vi "Meas Result Readings Panel.vi"(8 "error in":errorcluster, 11 "meas in":variant) -> (0 "error out":errorcluster, 3 "meas out":variant)   [LabVIEW 2020]
doc: "Panel for manual removal of readings."
uses:
  meas session.ctl
  Meas Sweep Config.ctl
  Meas Freq Info.ctl
  meas_swp_mode.ctl
  meas_sweep_flist_mode.ctl
  bridge/Bridge Session.ctl
  bridge/Bridge Type.ctl
  drivers/TWM client/TWM Session.ctl
  drivers/TWM client/TWM parameters.ctl
  drivers/TWM client/Meas Proc QWTB Uncertainty Mode.ctl
  bridge/Bridge Bias Session.ctl
  bridge/Bridge Bias Type.ctl
  bridge/Bridge Sim Mode.ctl
  source/Source Session.ctl
  source/Source Type.ctl
  drivers/AFG3101C/AFG3101C Session.ctl
  drivers/cDAQ DDS/cDAQ DDS Session.ctl
  drivers/cDAQ DDS/cDAQ DDS Setup.ctl
  drivers/cDAQ DDS/cDAQ DDS Timebase Mode.ctl
  drivers/Fluke 5XXX/top_lev/F5xxx_session.ctl
  drivers/Fluke 5XXX/top_lev/F5xxx_output_mode.ctl
  Meas Results Ref.ctl
  Meas Results.ctl
  bridge/Bridge Frequency Readings Data.ctl
  drivers/TWM client/Meas Proc QWTB Spectrum Data.ctl
  drivers/TWM client/TWM Phase Info.ctl
  Meas Result Major Format.ctl
  varilib/SGUI Assign References Mode.ctl
  <vilib>/Utility/miscctls.llb/LVRowAndColumnTypeDef.ctl
  varilib/varilib.lvlib
panel:
  in  "table xls":string[][](table) caption="Readings"
  in  "mnr fmt":T1=enum."%_5p" caption="Minor format"
  in  "mjr fmt":T1=enum."%_5p" caption="Major format"
  out "sweep spot index":u16
  out "phase index":u16
  in  "meas in":T2={"swp cfg"={"N"=0, "R"=0, "f list"=[], "smpl delay"=0.0, "set delay"=0.0, "set delay np"=0.0, "meas root"=path "", "meas name"="", "meas a-index"=FALSE, "rnd sweep"=FALSE, "mode"=enum."Frequency", "swp mode"=enum."Linear", "avg"=0, "subrec"=0, "multi-freq"=FALSE, "selfcal"=FALSE, "selfcal period [h]"=0.0}, "bridge"={"type"=enum."TWM client", "TWM"={"pipe name"="", "parameters"=[], "handle"=0, "fixed aper [s]"=0.0, "f-list [Hz]"=[], "discrete f-list"=FALSE, "unc mode"=enum."None", "unc mcc"=0, "unc first"=FALSE}, "last f"=0.0, "bias comp"={"bias type"=enum."dummy", "VISA"="", "Enable"=FALSE, "channel qu"=[], "channel Uinit"=[]}, "sim mode"=enum."Generic RLC network", "channel idns"=[], "sim phases"=1}, "src"={"type"=enum."Tektronix AFG3101C", "afg"={"VISA"="", "const"=0.0, "gen DC"=FALSE, "ext ref"=FALSE}, "cDAQ dds"={"device"="", "channels"=[], "mclk source"="", "mclk [Hz]"=0.0, "fs [Hz]"=0.0, "block [s]"=0.0, "buf [s]"=0.0, "task"="", "cmd queue"=refnum, "proc ref"=refnum, "smpl clock out"="/cDAQ3/PFI0", "export smpl clock"=FALSE, "DC ofs [V]"=[], "timebase source"="", "timebase mode"=enum."Local"}, "gain [V/A]"=1.0, "F5xxx session"={"VISA"="", "mode"=enum."AC voltage", "Earth on"=FALSE, "Ext ref lock"=FALSE}}, "results"=refnum} {"src"."cDAQ dds"."channels" min=0 step=1; "bridge"."TWM"."f-list [Hz]" format="%#_6p"; "swp cfg"."f list"."bias" format="%#_3p"; "swp cfg"."f list"."level" format="%#_3p"; "swp cfg"."f list"."fs [Hz]" format="%#_5p"; "swp cfg"."f list"."time [s]" format="%#_3p"; "swp cfg"."f list"."f/fs" format="%#_3p"; "swp cfg"."f list"."periods" format="%#_3f"; "swp cfg"."f list"."f [Hz]" format="%#_5p"}
  in  "btn rem":bool
  in  "rdgs ring spot":u16(ring) caption="Sweep spot selection" items=["Last measured"]
  in  "rdgs ring phase":u16(ring) caption="Phase selection"
  in  "btn ok":bool
  in  "table":string[][](table) caption="Readings (right click to show actions)"
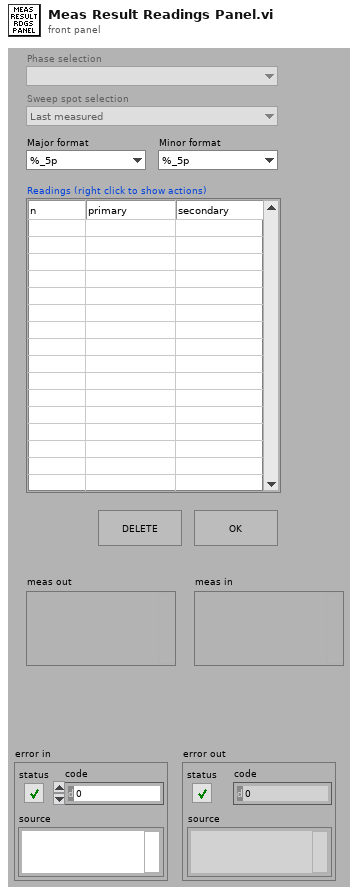
[diagram p1: front panel]
types:
  T1 = typedef "Meas Result Major Format.ctl" = enum16{"%_3p", "%_4p", "%_5p", "%_6p", "%_7p", "%_8p", "%_5f", "%_6f", "%_7f", "%_8f", "%_5e", "%_6e", "%_7e", "%_8e"}
  T2 = typedef "meas session.ctl" = cluster{"swp cfg":T3, "bridge":T7, "src":T15, "results":T22}
  T3 = typedef "Meas Sweep Config.ctl" = cluster{"N":i32, "R":i32, "f list":T4[], "smpl delay":dbl, "set delay":dbl, "set delay np":dbl, "meas root":path, "meas name":string, "meas a-index":bool, "rnd sweep":bool, "mode":T5, "swp mode":T6, "avg":i32, "subrec":i32, "multi-freq":bool, "selfcal":bool, "selfcal period [h]":dbl}
  T4 = typedef "Meas Freq Info.ctl" = cluster{"f [Hz]":dbl, "periods":dbl, "f/fs":dbl, "time [s]":dbl, "fs [Hz]":dbl, "N":i32, "level":dbl, "bias":dbl, "rdgs":i32, "f. id":i32}
  T5 = typedef "meas_swp_mode.ctl" = enum16{"Frequency", "Level", "Bias"}
  T6 = typedef "meas_sweep_flist_mode.ctl" = enum16{"Linear", "Log10"}
  T7 = typedef "Bridge Session.ctl" = cluster{"type":T8, "TWM":T9, "last f":dbl, "bias comp":T12, "sim mode":T14, "channel idns":string[], "sim phases":i32}
  T8 = typedef "Bridge Type.ctl" = enum16{"TWM client", "dummy"}
  T9 = typedef "TWM Session.ctl" = cluster{"pipe name":string, "parameters":T10[], "handle":i32, "fixed aper [s]":dbl, "f-list [Hz]":dbl[], "discrete f-list":bool, "unc mode":T11, "unc mcc":i32, "unc first":bool}
  T10 = typedef "TWM parameters.ctl" = cluster{"name":string, "value":string[]}
  T11 = typedef "Meas Proc QWTB Uncertainty Mode.ctl" = enum16{"None", "GUF", "Monte Carlo"}
  T12 = typedef "Bridge Bias Session.ctl" = cluster{"bias type":T13, "VISA":refnum<visa-resource-name>, "Enable":bool, "channel qu":string[], "channel Uinit":dbl[]}
  T13 = typedef "Bridge Bias Type.ctl" = enum16{"dummy", "CMI LiBbias V1.0"}
  T14 = typedef "Bridge Sim Mode.ctl" = enum16{"Generic RLC network", "Interchannel transfer"}
  T15 = typedef "Source Session.ctl" = cluster{"type":T16, "afg":T17, "cDAQ dds":T18, "gain [V/A]":dbl, "F5xxx session":T20}
  T16 = typedef "Source Type.ctl" = enum16{"Tektronix AFG3101C", "cDAQ DAC", "Fluke 5xxx", "Agilent 33120A", "dummy"}
  T17 = typedef "AFG3101C Session.ctl" = cluster{"VISA":refnum<visa-resource-name>, "const":dbl, "gen DC":bool, "ext ref":bool}
  T18 = typedef "cDAQ DDS Session.ctl" = cluster{"device":tag, "channels":i32[], "mclk source":tag, "mclk [Hz]":dbl, "fs [Hz]":dbl, "block [s]":dbl, "buf [s]":dbl, "task":refnum<k21>, "cmd queue":refnum<queue>, "proc ref":refnum<vi>, "smpl clock out":tag, "export smpl clock":bool, "DC ofs [V]":dbl[], "timebase source":tag, "timebase mode":T19}
  T19 = typedef "cDAQ DDS Timebase Mode.ctl" = enum16{"Local", "Take from ADC (e.g. NI 9238)", "Other source"}
  T20 = typedef "F5xxx_session.ctl" = cluster{"VISA":refnum<visa-resource-name>, "mode":T21, "Earth on":bool, "Ext ref lock":bool}
  T21 = typedef "F5xxx_output_mode.ctl" = enum16{"AC voltage", "AC current"}
  T22 = typedef "Meas Results Ref.ctl" = refnum<vi>
  T23 = typedef "varilib.lvlib/SGUI Assign References Mode.ctl" = enum16{"Add to stack", "Overwrite", "Release last", "Release ID"}
  T24 = typedef "LVRowAndColumnTypeDef.ctl" = cluster{"Row":i32, "Column":i32}
  T25 = typedef "Meas Results.ctl" = cluster{"freqs":T26[][], "locked":bool, "last fid":i32, "modified":bool, "mjr name":string, "mnr name":string, "last spectra":T27[][], "saved?":bool, "TWM phase":T28[], "time start":timestamp, "time stop":timestamp}
  T26 = typedef "Bridge Frequency Readings Data.ctl" = cluster{"Udut":dbl[], "Iref":dbl[], "Udc":dbl[], "Idc":dbl[], "mjr":dbl[], "mnr":dbl[], "mjr_sh":dbl[], "mnr_sh":dbl[], "u(mjr)":dbl[], "u(mnr)":dbl[], "ua2(mjr)":dbl[], "ua2(mnr)":dbl[], "n":i32, "f [Hz]":dbl, "fs [Hz]":dbl, "aperture [s]":dbl}
  T27 = typedef "Meas Proc QWTB Spectrum Data.ctl" = cluster{"x":sgl[], "y":sgl[], "label":string}
  T28 = typedef "TWM Phase Info.ctl" = cluster{"ref chn id (I)":string, "dut chn id (U)":string, "ref chn range [V]":dbl, "dut chn range [V]":dbl, "aperture [s]":dbl, "fs [Hz]":dbl, "ref chn transducer (I)":string, "dut chn transducer (U)":string}
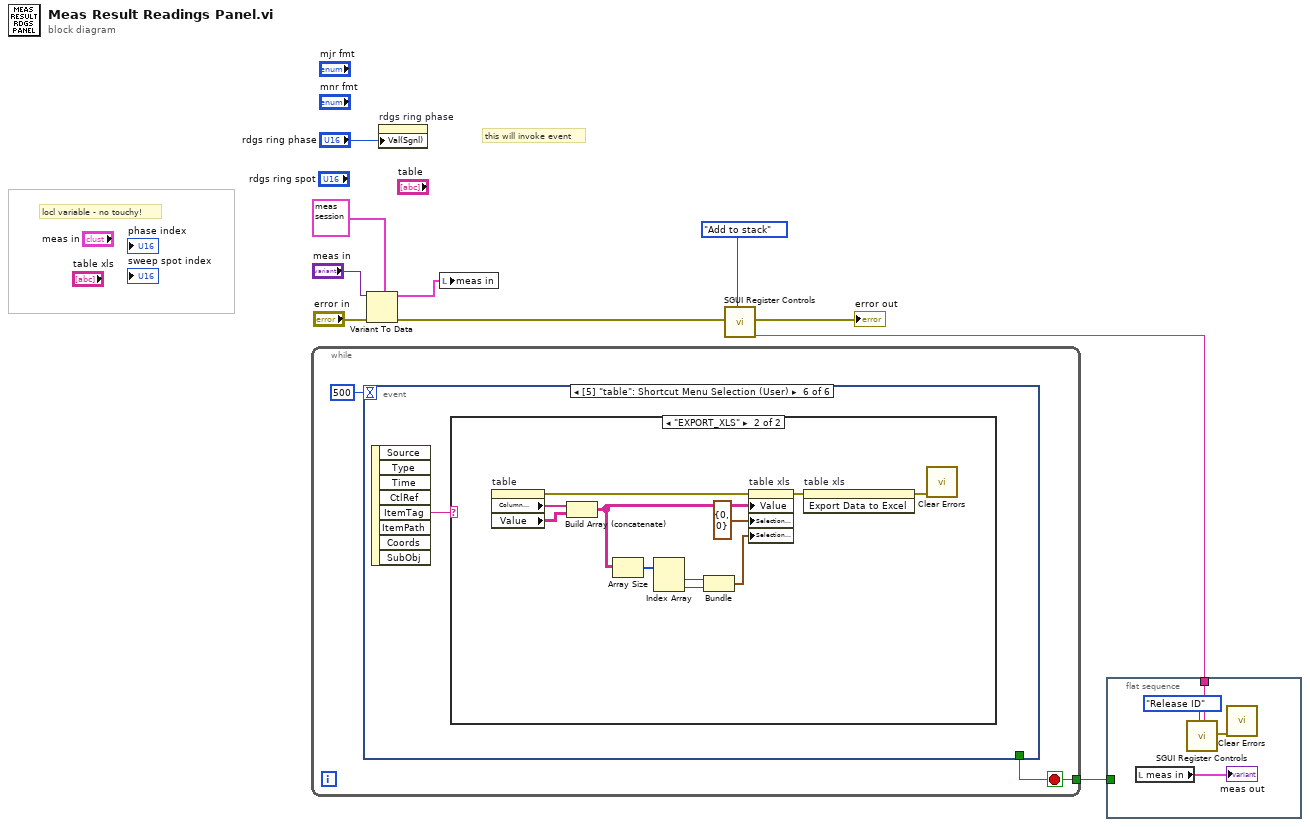
[diagram p0: block diagram]
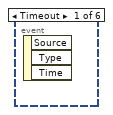
[diagram p2: hidden frame]
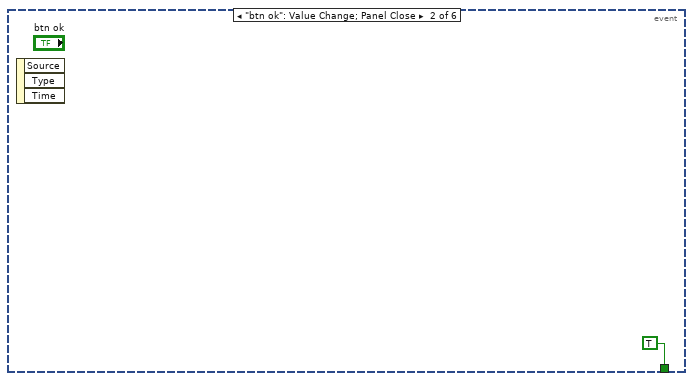
[diagram p3: hidden frame]
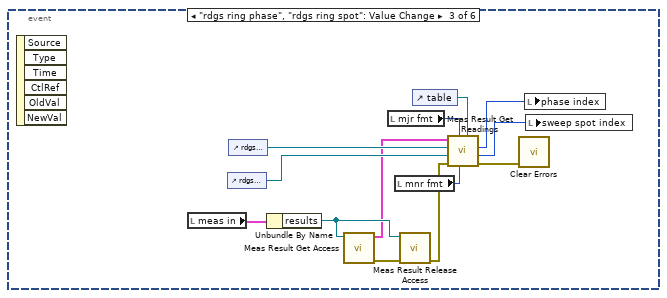
[diagram p4: hidden frame]
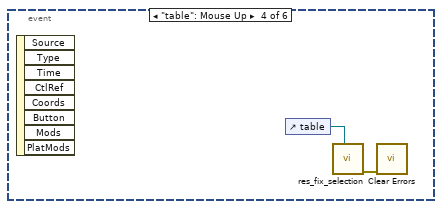
[diagram p5: hidden frame]
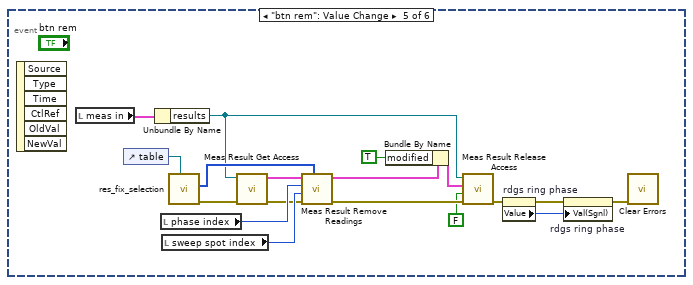
[diagram p6: hidden frame]
diagram:
  # "locl variable - no touchy!"
  # "this will invoke event"
  n1 = while {
    tunnel: [w12] -> w5
    stop <- w12 stop-if-true
    n2 = event shown="[5] \"table\": Shortcut Menu Selection (User)" {
      selector: _ -> [_ _ _ _ _ _]
      dyn-events: _ -> [_ _ _ _ _ _]
      timeout: 500 -> [_ _ _ _ _ _]
      tunnel: [_ TRUE _ _ _ _] -> w12
      event Timeout {
        n3 = event-data() -> ()  [unwired: 1 in, 3 out]
      }
      event "btn ok": Value Change; Panel Close {
        n4 = event-data() -> ()  [unwired: 1 in, 3 out]
      }
      event "rdgs ring phase", "rdgs ring spot": Value Change {
        n5 = event-data() -> ()  [unwired: 1 in, 6 out]
        n6 = local read "meas in"() -> (w22:T2)
        n7 = control-ref of="rdgs ring spot"() -> (w25:refnum<vi>)
        n8 = control-ref of="rdgs ring phase"() -> (w26:refnum<vi>)
        n9 = Unbundle By Name(w22) -> ("results"=w23:T22)
        n10 = call "Meas Result Get Access.vi"("results ref"=w23) -> ("error out"=w24:errorcluster, "results data"=w21:T25)  [unwired: 9 in]
        n11 = local read "mjr fmt"() -> (w15:T1)
        n12 = local read "mnr fmt"() -> (w14:T1)
        n13 = call "Meas Result Release Access.vi"("error in"=w24, "results ref"=w23) -> ("error out"=w19:errorcluster)  [unwired: 9 in]
        n14 = control-ref of="table"() -> (w20:refnum<vi>)
        n15 = call "Meas Result Get Readings.vi"("table ref"=w20, "mnr fmt"=w14, "mjr fmt"=w15, "error in (no error)"=w19, "ring spot"=w25, "ring phase"=w26, "result"=w21) -> ("error out"=w18:errorcluster, "sweep spot index"=w16:u16, "phase index"=w17:u16)  [unwired: 2 out]
        n16 = call <vilib>:"Clear Errors.vi"("error in (no error)"=w18) -> ()  [unwired: 5 in, 2 out]
        n17 = local write "phase index"(w17) -> ()
        n18 = local write "sweep spot index"(w16) -> ()
      }
      event "table": Mouse Up {
        n19 = event-data() -> ()  [unwired: 1 in, 8 out]
        n20 = control-ref of="table"() -> (w28:refnum<vi>)
        n21 = call "res_fix_selection.vi"("list"=w28) -> ("error out"=w27:errorcluster)  [unwired: 8 in, 2 out]
        n22 = call <vilib>:"Clear Errors.vi"("error in (no error)"=w27) -> ()  [unwired: 5 in, 2 out]
      }
      event "btn rem": Value Change {
        n23 = event-data() -> ()  [unwired: 1 in, 6 out]
        n24 = local read "meas in"() -> (w39:T2)
        n25 = control-ref of="table"() -> (w40:refnum<vi>)
        n26 = Unbundle By Name(w39) -> ("results"=w37:T22)
        n27 = local read "phase index"() -> (w46:u16)
        n28 = local read "sweep spot index"() -> (w45:u16)
        n29 = call "res_fix_selection.vi"("list"=w40) -> ("error out"=w44:errorcluster, "ids of selected"=w38:i32[])  [unwired: 8 in, 1 out]
        n30 = call "Meas Result Get Access.vi"("error in"=w44, "results ref"=w37) -> ("error out"=w43:errorcluster, "results data"=w42:T25)  [unwired: 8 in]
        n31 = call "Meas Result Remove Readings.vi"("ids of selected"=w38, "error in"=w43, "sweep spot index"=w45, "phase index"=w46, "result"=w42) -> ("error out"=w41:errorcluster, "result out"=w31:T25)  [unwired: 5 in]
        n32 = Bundle By Name(cluster=w31, "modified"=TRUE) -> (w30:T25)
        n33 = call "Meas Result Release Access.vi"("error in"=w41, "Release only (True)"=FALSE, "results data in"=w30, "results ref"=w37) -> ("error out"=w35:errorcluster)  [unwired: 7 in]
        n34 = property on="rdgs ring phase" class="Ring (strict)"(error in=w35) -> (error out=w33:errorcluster, "Value"=w34:u16)  [unwired: 1 in, 1 out]
        n35 = property on="rdgs ring phase" class="Ring (strict)"(error in=w33, "Val(Sgnl)"=w34) -> (error out=w32:errorcluster)  [unwired: 1 in, 1 out]
        n36 = call <vilib>:"Clear Errors.vi"("error in (no error)"=w32) -> ()  [unwired: 5 in, 2 out]
      }
      event "table": Shortcut Menu Selection (User) {
        n37 = event-data() -> ("ItemTag"=w47:string)  [unwired: 1 in, 7 out]
        n38 = case shown="\"EXPORT_XLS\"" w47 {
          frame "False", Default {
          }
          frame "EXPORT_XLS" {
            n39 = property on="table" class="Tbl (strict)"() -> (error out=w55:errorcluster, "Column Headers[]"=w57:string[], "Value"=w56:string[][])  [unwired: 2 in, 1 out]
            n40 = Build Array (concatenate)(w57, w56) -> (w54:string[][])
            n41 = Array Size(array=w54) -> (size(s)=w58:i32[])
            n42 = Index Array(array=w58) -> (element #1=w51:i32, element #2=w52:i32)  [unwired: 2 in]
            n43 = Bundle(w51, w52) -> (w50:cluster{i32, i32})  [unwired: 1 in]
            n44 = property on="table xls" class="Tbl (strict)"(error in=w55, "Value"=w54, "Selection Start"=T24 {"Row"=0, "Column"=0}, "Selection Size"=w50) -> (error out=w49:errorcluster)  [unwired: 1 in, 1 out]
            n45 = invoke on="table xls" class="Tbl (strict)" method="Export Data to Excel"(error in=w49) -> (error out=w48:errorcluster)  [unwired: 2 in, 2 out]
            n46 = call <vilib>:"Clear Errors.vi"("error in (no error)"=w48) -> ()  [unwired: 5 in, 2 out]
          }
        }
      }
    }
  }
  n47 = Variant To Data(error in="error in", type=T2 {"swp cfg"={"N"=0, "R"=0, "f list"=[], "smpl delay"=0.0, "set delay"=0.0, "set delay np"=0.0, "meas root"=path "", "meas name"="", "meas a-index"=FALSE, "rnd sweep"=FALSE, "mode"=enum."Frequency", "swp mode"=enum."Linear", "avg"=0, "subrec"=0, "multi-freq"=FALSE, "selfcal"=FALSE, "selfcal period [h]"=0.0}, "bridge"={"type"=enum."TWM client", "TWM"={"pipe name"="", "parameters"=[], "handle"=0, "fixed aper [s]"=0.0, "f-list [Hz]"=[], "discrete f-list"=FALSE, "unc mode"=enum."None", "unc mcc"=0, "unc first"=FALSE}, "last f"=0.0, "bias comp"={"bias type"=enum."dummy", "VISA"="", "Enable"=FALSE, "channel qu"=[], "channel Uinit"=[]}, "sim mode"=enum."Generic RLC network", "channel idns"=[], "sim phases"=1}, "src"={"type"=enum."Tektronix AFG3101C", "afg"={"VISA"="", "const"=0.0, "gen DC"=FALSE, "ext ref"=FALSE}, "cDAQ dds"={"device"="", "channels"=[], "mclk source"="", "mclk [Hz]"=0.0, "fs [Hz]"=0.0, "block [s]"=0.0, "buf [s]"=0.0, "task"="", "cmd queue"=refnum, "proc ref"=refnum, "smpl clock out"="/cDAQ3/PFI0", "export smpl clock"=FALSE, "DC ofs [V]"=[], "timebase source"="", "timebase mode"=enum."Local"}, "gain [V/A]"=1.0, "F5xxx session"={"VISA"="", "mode"=enum."AC voltage", "Earth on"=FALSE, "Ext ref lock"=FALSE}}, "results"=refnum} ("meas in"), Variant="meas in") -> (data=w6:T2, error out=w1:errorcluster)
  n48 = property on="rdgs ring phase" class="Ring (strict)"("Val(Sgnl)"="rdgs ring phase") -> ()  [unwired: 2 in, 2 out]
  n49 = local write "meas in"(w6) -> ()
  n50 = call "SGUI Register Controls.vi"("error in"=w1, "register mode (overwrite)"=SGUI_Assign_References_Mode."Add to stack") -> ("assigned ID"=w2:string, "error out"=→"error out":errorcluster)  [unwired: 15 in, 1 out]
  n51 = flat-sequence {
    tunnel: w5 -> [_]
    tunnel: w2 -> [w61]
    frame #0 {
      n52 = local read "meas in"() -> (→"meas out":T2)
      n53 = call "SGUI Register Controls.vi"("register mode (overwrite)"=SGUI_Assign_References_Mode."Release ID", "controls ID (empty)"=w61) -> ("error out"=w60:errorcluster)  [unwired: 15 in, 2 out]
      n54 = call <vilib>:"Clear Errors.vi"("error in (no error)"=w60) -> ()  [unwired: 5 in, 2 out]
    }
  }
